vi "Database Import Value.vi"(6 "data":variant, 8 "error in (no error)":errorcluster, 9 "columns":string[](array[string]), 10 "table":string, 11 "object in":refnum<class "DatabaseAPI.lvclass">) -> (0 "error out":errorcluster, 3 "object out":refnum<class "DatabaseAPI.lvclass">)   [LabVIEW 2015, in "DatabaseAPI.lvclass"]
uses:
  DatabaseAPI.lvclass
  DatabaseAPI.lvclass/DatabaseAPI.ctl
  <vilib>/addons/database/Connection.llb/DB Tools Open Connec (String).vi
  <vilib>/addons/database/NI_Database_API.lvlib
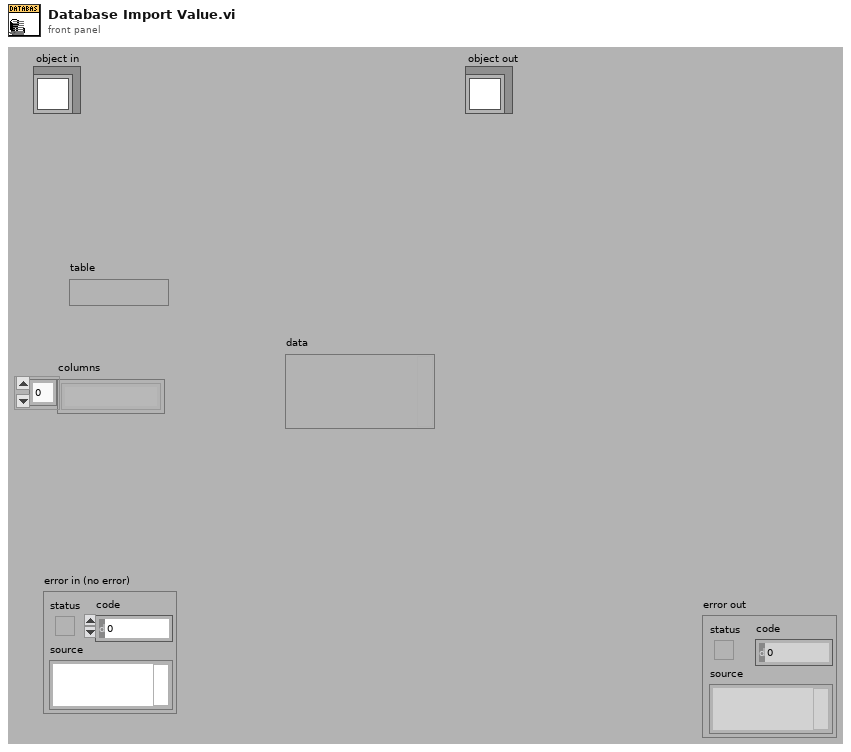
[diagram p1: front panel]
types:
  T1 = typedef "NI_Database_API.lvlib/Conn ObjectReference.ctl" = refnum<k1>
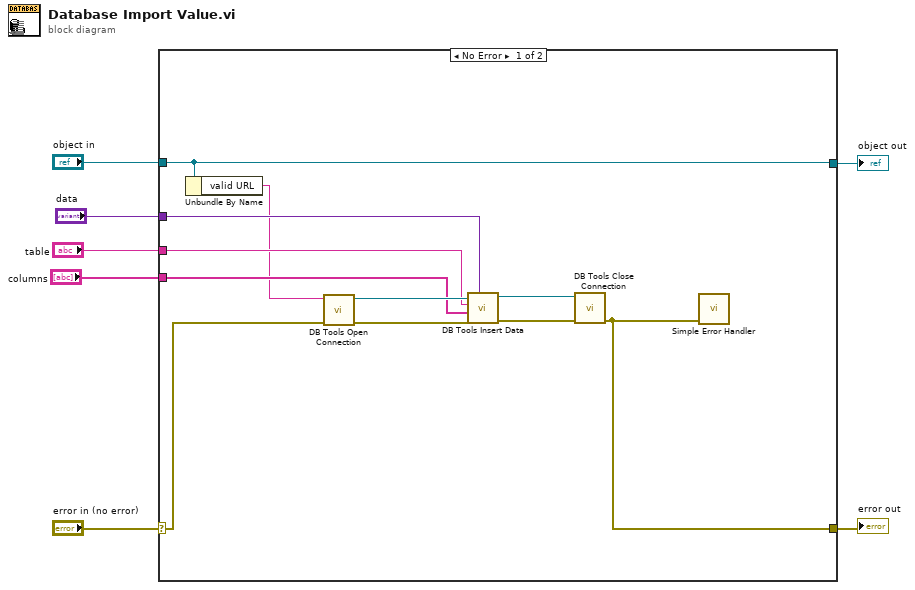
[diagram p0: block diagram]
diagram:
  n1 = case shown="No Error" "error in (no error)" {
    selector: "error in (no error)" -> [w11 w20]
    tunnel: [w10 w20] -> w6
    tunnel: [w9 w19] -> w4
    tunnel: "object in" -> [w9 w19]
    tunnel: "table" -> [w16 _]
    tunnel: "columns" -> [w15 _]
    tunnel: "data" -> [w14 _]
    frame No Error {
      n2 = Unbundle By Name(w9) -> ("valid URL"=w8:string)
      n3 = call-poly <vilib>:"DB Tools Open Connection.vi"("error in (no error)"=w11, "connection information"=w8) -> ("error out"=w17:errorcluster, "connection reference"=w18:T1)  [unwired: 6 in]
      n4 = call <vilib>:"DB Tools Insert Data.vi"("data"=w14, "error in (no error)"=w17, "columns"=w15, "table"=w16, "connection reference"=w18) -> ("error out"=w12:errorcluster, "connection reference out"=w13:T1)  [unwired: 5 in]
      n5 = call <vilib>:"DB Tools Close Connection.vi"("error in (no error)"=w12, "connection reference"=w13) -> ("error out"=w10:errorcluster)  [unwired: 5 in]
      n6 = call <vilib>:"Simple Error Handler.vi"("error in (no error)"=w10) -> ()  [unwired: 4 in, 5 out]
    }
    frame Error {
    }
  }
  "error out" <- w6
  "object out" <- w4
